vi "LoadPatientDateInfo_Palpation-Kamronn-Medtech.vi"(8 "error in":errorcluster, 11 "File path":path) -> (0 "error out":errorcluster, 3 "palpation":cluster{"right":string, "left":string})   [LabVIEW 2013, in "main.lvlib"]
uses:
  main.lvlib
  Controls/date_specific_info.ctl
  Globals/DataPathGlobalVariable.vi
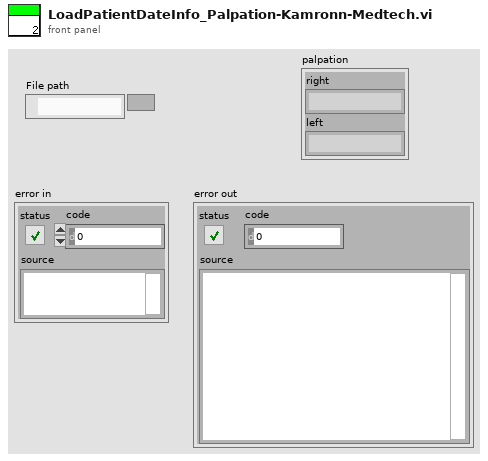
[diagram p1: front panel]
types:
  T1 = typedef "main.lvlib/date_specific_info.ctl" = cluster{"profile":cluster{"id":string, "name":string, "operator":string, "doctor":string, "comment":string}, "hospital":cluster{"name":string, "department":string, "address":string}, "palpation":cluster{"right":string, "left":string}, "Armpressure Right":cluster{"sys":dbl, "dia":dbl, "puls":dbl, "date":string, "time":string, "code":string, "serial":string, "temp":dbl, "activity":string}[], "Armpressure Left":cluster{"sys":dbl, "dia":dbl, "puls":dbl, "date":string, "time":string, "code":string, "serial":string, "temp":dbl, "activity":string}[]}
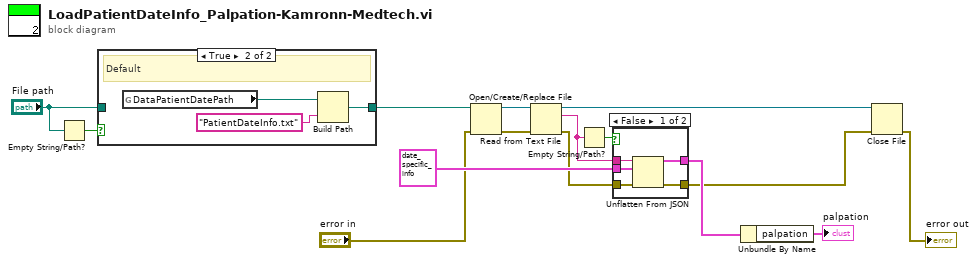
[diagram p0: block diagram]
diagram:
  n1 = Empty String/Path?(string/path="File path") -> (empty?=w3:bool)
  n2 = case shown="True" w3 {
    tunnel: [w16 w17] -> w1
    tunnel: "File path" -> [w16 _]
    frame False {
    }
    frame True {
      # "Default"
      n3 = global read "DataPathGlobalVariable.vi" "DataPatientDatePath"() -> (w19:path)
      n4 = Build Path(base path=w19, name or relative path="PatientDateInfo.txt") -> (appended path=w17:path)
    }
  }
  n5 = Open/Create/Replace File(file path (use dialog)=w1, error in="error in") -> (refnum out=w7:refnum<file>, error out=w6:errorcluster)  [unwired: 4 in, 1 out]
  n6 = Read from Text File(file (use dialog)=w7, error in=w6) -> (refnum out=w11:refnum<file>, text=w9:string, error out=w14:errorcluster)  [unwired: 2 in, 1 out]
  n7 = Empty String/Path?(string/path=w9) -> (empty?=w8:bool)
  n8 = case shown="False" w8 {
    tunnel: T1 {"profile"={"id"="", "name"="", "operator"="", "doctor"="", "comment"=""}, "hospital"={"name"="", "department"="", "address"=""}, "palpation"={"right"="", "left"=""}, "Armpressure Right"=[], "Armpressure Left"=[]} ("date_specific_info") -> [w24 w25]
    tunnel: w14 -> [w23 w26]
    tunnel: [w22 w25] -> w12
    tunnel: [w21 w26] -> w10
    tunnel: w9 -> [w20 _]
    frame False {
      n9 = Unflatten From JSON(JSON string=w20, type and defaults=w24, error in (no error)=w23) -> (value=w22:T1, error out=w21:errorcluster)  [unwired: 4 in]
    }
    frame True {
    }
  }
  n10 = Unbundle By Name(w12) -> ("palpation"=→"palpation":cluster{"right":string, "left":string})
  n11 = Close File(refnum=w11, error in=w10) -> (error out=→"error out":errorcluster)  [unwired: 1 out]
